vi "Joystick Global.vi"() -> ()   [LabVIEW 2013]
panel:
  in  "Cluster 2":cluster{}
  out "Cluster":T1
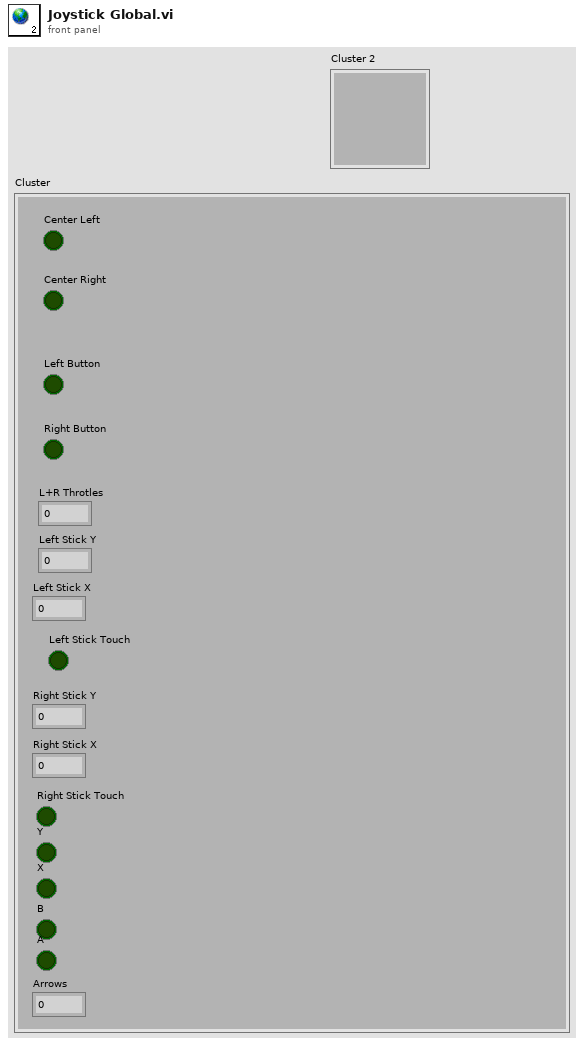
[diagram p1: front panel]
types:
  T1 = cluster{"Center Left":bool, "Center Right":bool, "Left Button":bool, "Right Button":bool, "L+R Throtles":dbl, "Left Stick Y":dbl, "Left Stick X":dbl, "Left Stick Touch":bool, "Right Stick Y":dbl, "Right Stick X":dbl, "Right Stick Touch":bool, "Y":bool, "X":bool, "B":bool, "A":bool, "Arrows":dbl}
diagram:
